vi "zmq REP.vi"() -> ()   [LabVIEW 2015]
uses:
  <vilib>/addons/zeromq/poll_event_data.ctl
  <vilib>/addons/zeromq/socket_type.ctl
  <vilib>/addons/zeromq/zeromq.lvlib
  <vilib>/addons/zeromq/zmq_context.lvclass
  <vilib>/addons/zeromq/zmq_socket.lvclass
panel:
  out "h":bool
  out "data":string
  out "identity":string
  out "error out":errorcluster
  in  "Stop":bool
  in  "ZMQ endpoint":string="tcp://127.0.0.1:5555"
  # "*:5555"
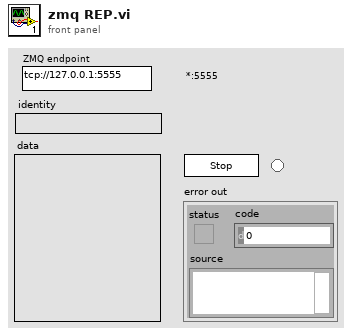
[diagram p1: front panel]
types:
  T1 = typedef "zeromq.lvlib/socket_type.ctl" = enum8{"ZMQ_PAIR", "ZMQ_PUB", "ZMQ_SUB", "ZMQ_REQ", "ZMQ_REP", "ZMQ_DEALER", "ZMQ_ROUTER", "ZMQ_PULL", "ZMQ_PUSH", "ZMQ_XPUB", "ZMQ_XSUB"}
  T2 = typedef "zeromq.lvlib/poll_event_data.ctl" = cluster{"identity":string, "data":string[]}
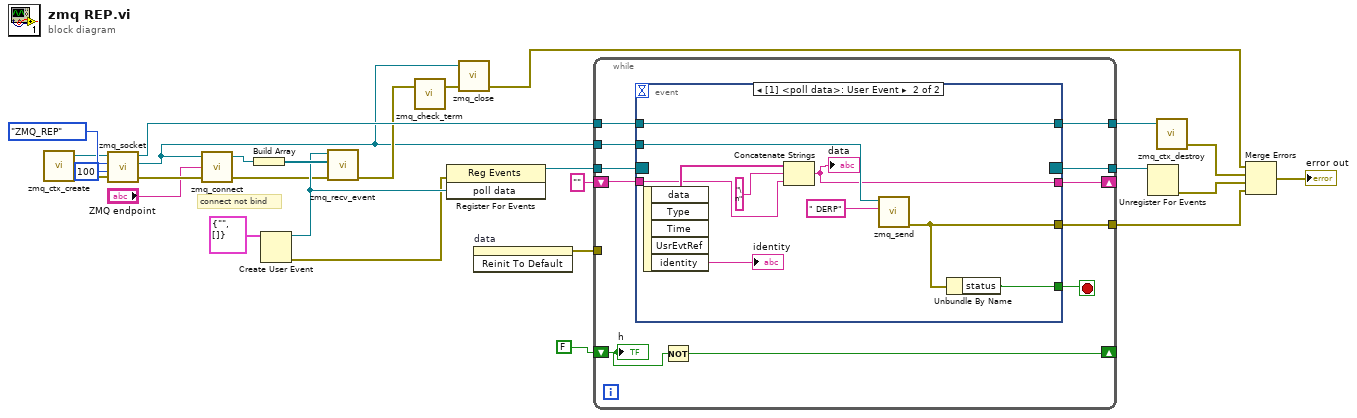
[diagram p0: block diagram]
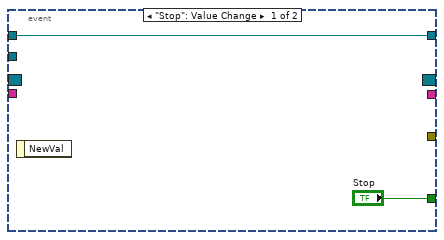
[diagram p2: hidden frame]
diagram:
  # "connect not bind"
  n1 = call <vilib>:"zmq_ctx_create.vi"() -> ("error out"=w25:errorcluster, "context out"=w12:refnum<class "zmq_context.lvclass">)  [unwired: 4 in]
  n2 = call <vilib>:"zmq_socket.vi"("error in"=w25, "linger (ms)"=100, "socket type"=socket_type."ZMQ_REP", "context in"=w12) -> ("error out"=w23:errorcluster, "socket out"=w15:refnum<class "zmq_socket.lvclass">, "context out"=w20:refnum<class "zmq_context.lvclass">)  [unwired: 1 in]
  n3 = call <vilib>:"zmq_connect.vi"("error in"=w23, "endpoint"="ZMQ endpoint", "socket in"=w15) -> ("error out"=w13:errorcluster, "socket out"=w22:refnum<class "zmq_socket.lvclass">)  [unwired: 1 in]
  n4 = Build Array(w22) -> (w21:refnum<class "zmq_socket.lvclass">[])
  n5 = Create User Event(user event datatype=T2 {"identity"="", "data"=[]} ("poll data")) -> (user event=w19:refnum<user-event>, error out=w16:errorcluster)  [unwired: 1 in]
  n6 = call <vilib>:"zmq_recv_event.vi"("error in"=w13, "sockets"=w21, "poll event"=w19) -> ("error out"=w17:errorcluster)  [unwired: 3 in, 1 out]
  n7 = call <vilib>:"zmq_check_term.vi"("error in"=w17) -> ("error out"=w27:errorcluster)  [unwired: 1 in, 1 out]
  n8 = register-events(error in=w16, w19) -> (reference out=w18:refnum<event-registration>)  [unwired: 1 in, 1 out]
  n9 = call <vilib>:"zmq_close.vi"("error in"=w27, "socket"=w15) -> ("error out"=w5:errorcluster)  [unwired: 3 in]
  n10 = invoke on="data" class="Str" method="Reinit To Default"() -> (error out=w3:errorcluster)  [unwired: 3 in, 2 out]
  n11 = while {
    tunnel: w20 -> [w37]
    tunnel: w18 -> [w36]
    tunnel: w15 -> [w35]
    tunnel: [w34] -> w14
    shift-right: [w32] -> _
    shift-left: "" -> [w31]
    tunnel: [w33] -> w10
    tunnel: [w30] -> w4
    tunnel: w3 -> [_]
    shift-right: [w28] -> _
    shift-left: FALSE ("Stop") -> [w29]
    stop <- w38 stop-if-true
    n12 = event shown="[1] <poll data>: User Event" {
      selector: w36 -> [_ _]
      dyn-events: [_ _] -> w33
      timeout: _ -> [_ _]
      tunnel: ["Stop" w47] -> w38
      tunnel: w37 -> [w39 w46]
      tunnel: w35 -> [_ w49]
      tunnel: [w39 w46] -> w34
      tunnel: [_ w43] -> w32
      tunnel: w31 -> [_ w42]
      tunnel: [_ w41] -> w30
      event "Stop": Value Change {
        n13 = event-data() -> ()  [unwired: 1 in, 1 out]
      }
      event User Event {
        n14 = event-data() -> ("data"=w45:string[], "identity"=→"identity":string)  [unwired: 1 in, 3 out]
        n15 = Concatenate Strings(w45, "\n" ("String"), w42) -> (w43:string)
        "data" <- w43
        n16 = call <vilib>:"zmq_send.vi"("data"=" DERP", "socket in"=w49) -> ("error out"=w41:errorcluster)  [unwired: 5 in, 1 out]
        n17 = Unbundle By Name(w41) -> ("status"=w47:bool)
      }
    }
    n18 = Not(x=w29) -> (.not. x?=w28:bool)
    "h" <- w29
  }
  n19 = Unregister For Events(event registration refnum=w10) -> (error out=w7:errorcluster)  [unwired: 1 in]
  n20 = call <vilib>:"zmq_ctx_destroy.vi"("context in"=w14) -> ("error out"=w8:errorcluster)  [unwired: 4 in]
  n21 = Merge Errors(w5, w8, w7, w4) -> (→"error out":errorcluster)
